vi "U8ToU32.vi"(8 "x 4":u8, 9 "x 3":u8, 10 "x 2":u8, 11 "x":u8) -> (2 "result":u32)   [LabVIEW 2013]
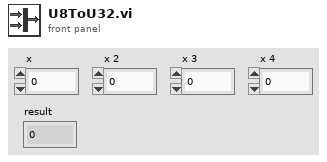
[diagram p1: front panel]
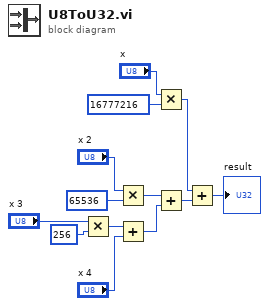
[diagram p0: block diagram]
diagram:
  n1 = Multiply(x="x 3", y=u32 256) -> (x*y=w9:u32)
  n2 = Multiply(x="x 2", y=u32 65536) -> (x*y=w12:u32)
  n3 = Add(x=w9, y="x 4") -> (x+y=w11:u32)
  n4 = Multiply(x="x", y=u32 16777216) -> (x*y=w3:u32)
  n5 = Add(x=w12, y=w11) -> (x+y=w2:u32)
  n6 = Add(x=w3, y=w2) -> (x+y=→"result":u32)
